vi "MathFinder_Case-Power.vi"(0 "Whole Match":string, 7 "After Match":string, 11 "error in (no error)":errorcluster) -> (4 "in1":string, 6 "Expression":string, 8 "in2":string, 15 "error out":errorcluster)   [LabVIEW 2014]
uses:
  <vilib>/regexp/Match Regular Expression.xnode
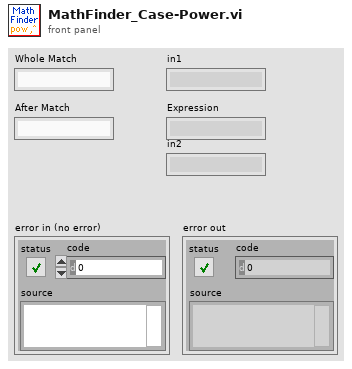
[diagram p1: front panel]
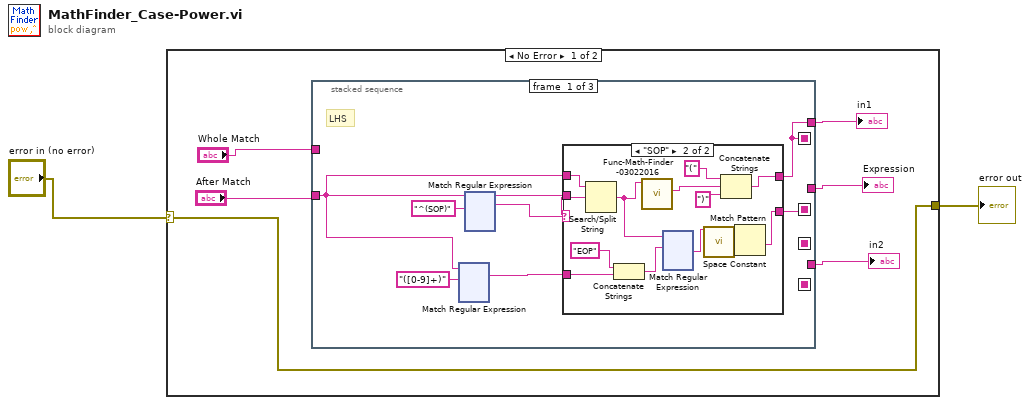
[diagram p0: block diagram]
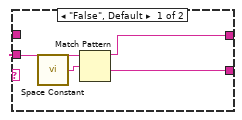
[diagram p2: hidden frame]
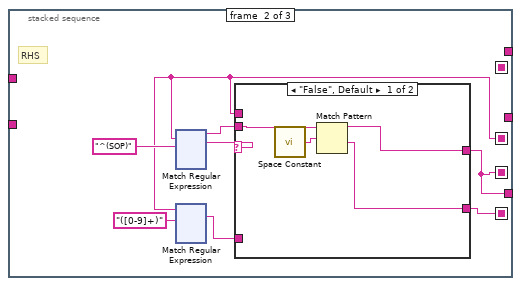
[diagram p3: hidden frame]
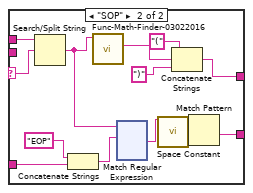
[diagram p4: hidden frame]
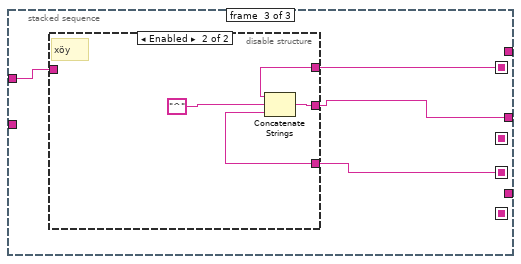
[diagram p5: hidden frame]
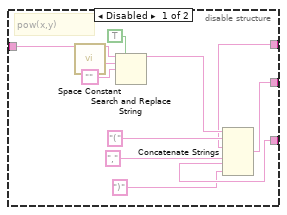
[diagram p6: hidden frame]
diagram:
  n1 = case shown="No Error" "error in (no error)" {
    selector: "error in (no error)" -> [w3 w762]
    tunnel: [w3 w762] -> w1
    frame No Error {
      n2 = stacked-sequence {
        seq-local: [w14 _ _] -> [_ w378 _]
        seq-local: [_ w380 _] -> [_ _ w745]
        seq-local: [w13 _ _] -> [_ _ w746]
        seq-local: [_ w376 _] -> [_ _ _]
        tunnel: [_ _ w744] -> w4
        tunnel: [_ w380 _] -> w5
        tunnel: [w13 _ _] -> w6
        tunnel: "Whole Match" -> [_ _ w743]
        tunnel: "After Match" -> [w9 _ _]
        frame #0 {
          # "LHS"
          n3 = xnode "Match Regular Expression"("input string"=w9, "regular expression"="([0-9]+)") -> ("whole match"=w10:string)  [unwired: 4 in, 4 out]
          n4 = xnode "Match Regular Expression"("input string"=w9, "regular expression"="^(SOP)") -> ("before match"=w15:string, "whole match"=w12:string)  [unwired: 4 in, 3 out]
          n5 = case shown="\"SOP\"" w12 {
            selector: w12 -> [_ w147]
            tunnel: w15 -> [w134 _]
            tunnel: [w132 w140] -> w14
            tunnel: [w131 w136] -> w13
            tunnel: w10 -> [_ w145]
            tunnel: w9 -> [_ w135]
            frame "False", Default {
              n6 = call <vilib>:"Space Constant.vi"() -> ("String"=w133:string)
              n7 = Match Pattern(string=w134, regular expression=w133) -> (before substring=w131:string, after substring=w132:string)  [unwired: 1 in, 2 out]
            }
            frame "SOP" {
              n8 = Search/Split String(string=w135, search string/char (-)=w147) -> (match + rest of string=w143:string)  [unwired: 1 in, 2 out]
              n9 = Concatenate Strings("EOP" ("regular expression"), w145) -> (w144:string)
              n10 = call "Func-Math-Finder-03022016.vi"("Get Tagged String"=w143) -> ("Expression"=w137:string)  [unwired: 8 in, 2 out]
              n11 = xnode "Match Regular Expression"("input string"=w143, "regular expression"=w144) -> ("after match"=w141:string)  [unwired: 4 in, 4 out]
              n12 = call <vilib>:"Space Constant.vi"() -> ("String"=w142:string)
              n13 = Concatenate Strings("(" ("string"), w137, ")" ("string")) -> (w136:string)
              n14 = Match Pattern(string=w141, regular expression=w142) -> (after substring=w140:string)  [unwired: 1 in, 3 out]
            }
          }
        }
        frame #1 {
          # "RHS"
          n15 = xnode "Match Regular Expression"("input string"=w378, "regular expression"="^(SOP)") -> ("before match"=w381:string, "whole match"=w382:string)  [unwired: 4 in, 3 out]
          n16 = xnode "Match Regular Expression"("input string"=w378, "regular expression"="([0-9]+)") -> ("whole match"=w377:string)  [unwired: 4 in, 4 out]
          n17 = case shown="\"False\", Default" w382 {
            selector: w382 -> [_ w513]
            tunnel: w381 -> [w501 _]
            tunnel: [w499 w510] -> w380
            tunnel: w378 -> [_ w514]
            tunnel: w377 -> [_ w504]
            tunnel: [w498 w502] -> w376
            frame "False", Default {
              n18 = call <vilib>:"Space Constant.vi"() -> ("String"=w500:string)
              n19 = Match Pattern(string=w501, regular expression=w500) -> (before substring=w499:string, after substring=w498:string)  [unwired: 1 in, 2 out]
            }
            frame "SOP" {
              n20 = Search/Split String(string=w514, search string/char (-)=w513) -> (match + rest of string=w503:string)  [unwired: 1 in, 2 out]
              n21 = Concatenate Strings("EOP" ("regular expression"), w504) -> (w506:string)
              n22 = call "Func-Math-Finder-03022016.vi"("Get Tagged String"=w503) -> ("Expression"=w509:string)  [unwired: 8 in, 2 out]
              n23 = xnode "Match Regular Expression"("input string"=w503, "regular expression"=w506) -> ("after match"=w508:string)  [unwired: 4 in, 4 out]
              n24 = call <vilib>:"Space Constant.vi"() -> ("String"=w505:string)
              n25 = Concatenate Strings("(" ("string"), w509, ")" ("string")) -> (w510:string)
              n26 = Match Pattern(string=w508, regular expression=w505) -> (after substring=w502:string)  [unwired: 1 in, 3 out]
            }
          }
        }
        frame #2 {
          n27 = disable-structure shown="Enabled" {
            disable-tunnel: w743 -> [w751 _]
            disable-tunnel: [w750 w760] -> w744
            disable-tunnel: w746 -> [w748 w759]
            disable-tunnel: w745 -> [w749 w758]
            frame Disabled {
              # "pow(x,y)"
              n28 = call <vilib>:"Space Constant.vi"() -> ("String"=w755:string)
              n29 = Search and Replace String(replace all?=TRUE ("replace all? (F)"), input string=w751, search string=w755, replace string="" ("string")) -> (result string=w756:string)  [unwired: 4 in, 3 out]
              n30 = Concatenate Strings(w756, "(" ("string"), w748, "," ("string"), w749, ")" ("string")) -> (w750:string)
            }
            frame Enabled {
              # "xöy"
              n31 = Concatenate Strings(w759, "^" ("string"), w758) -> (w760:string)
            }
          }
        }
      }
      "in1" <- w6
      "Expression" <- w4
      "in2" <- w5
    }
    frame Error {
    }
  }
  "error out" <- w1
